vi "Queue Dequeue.vi"(8 "Error In":errorcluster, 11 "Queue In":refnum<queue>) -> (0 "Error Out":errorcluster, 1 "Data":variant, 3 "State":string)   [LabVIEW 2015]
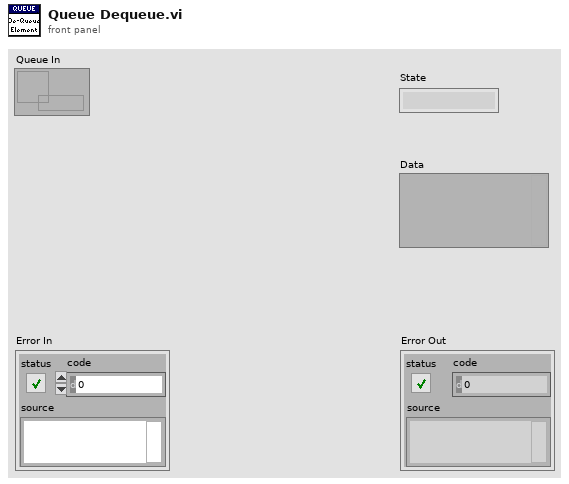
[diagram p1: front panel]
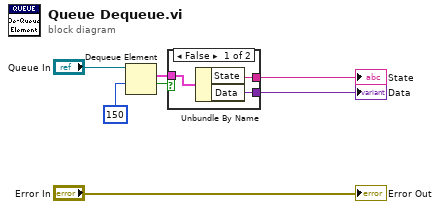
[diagram p0: block diagram]
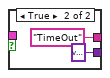
[diagram p2: hidden frame]
diagram:
  n1 = Dequeue Element(queue="Queue In", timeout in ms (-1)=150) -> (element=w6:cluster{"State":string, "Data":variant}, timed out?=w5:bool)  [unwired: 1 in, 2 out]
  n2 = case shown="False" w5 {
    tunnel: w6 -> [w10 _]
    tunnel: [w9 variant ("Data")] -> w2
    tunnel: [w8 "TimeOut" ("State")] -> w3
    frame False {
      n3 = Unbundle By Name(w10) -> ("State"=w8:string, "Data"=w9:variant)
    }
    frame True {
    }
  }
  "State" <- w3
  "Data" <- w2
  "Error Out" <- "Error In"
